vi "Reset.vi"(8 "error in (no error)":errorcluster, 11 "Vector in":refnum<class "Vector Parent.lvclass">) -> (0 "error out":errorcluster, 3 "Vector out":refnum<class "Vector Parent.lvclass">)   [LabVIEW 2019, in "Vector Parent.lvclass"]
uses:
  Vector Parent.lvclass
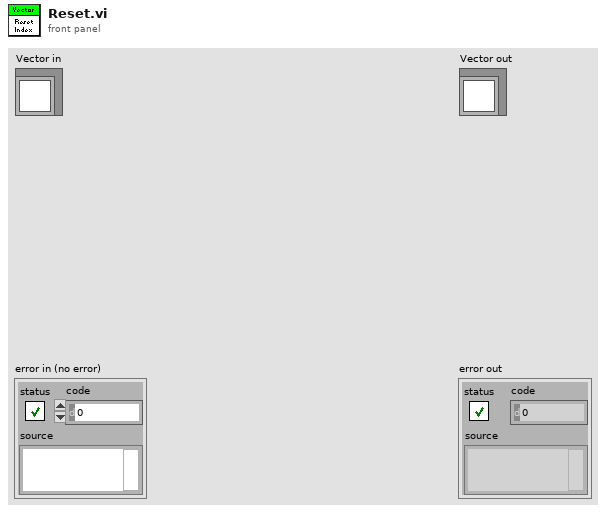
[diagram p1: front panel]
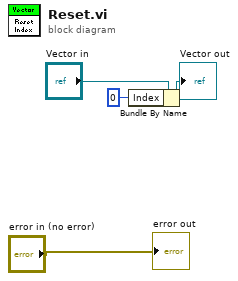
[diagram p0: block diagram]
diagram:
  n1 = Bundle By Name(cluster="Vector in", "Index"=0) -> (→"Vector out":refnum<class "Vector Parent.lvclass">)
  "error out" <- "error in (no error)"
